vi "Joystick_Globals.vi"() -> ()   [LabVIEW 2019]
panel:
  in  "Joystick_2":string="Joystick_2"
  in  "Joystick_1":string="Joystick_1"
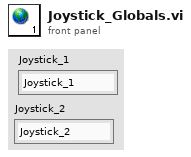
[diagram p1: front panel]
diagram:
